vi "Handle Command.vi"(8 "error in (no error)":errorcluster, 9 "Data":variant, 10 "Command":string, 11 "Instrument in":refnum<class "Instrument.lvclass">) -> (0 "error out":errorcluster, 1 "Processed Data":variant, 2 "Command":string, 3 "Instrument out":refnum<class "Instrument.lvclass">)   [LabVIEW 2016, in "Instrument.lvclass"]
uses:
  Instrument.lvclass
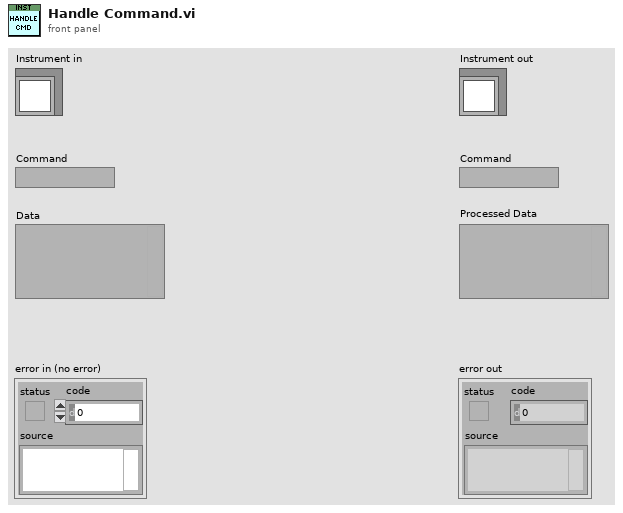
[diagram p1: front panel]
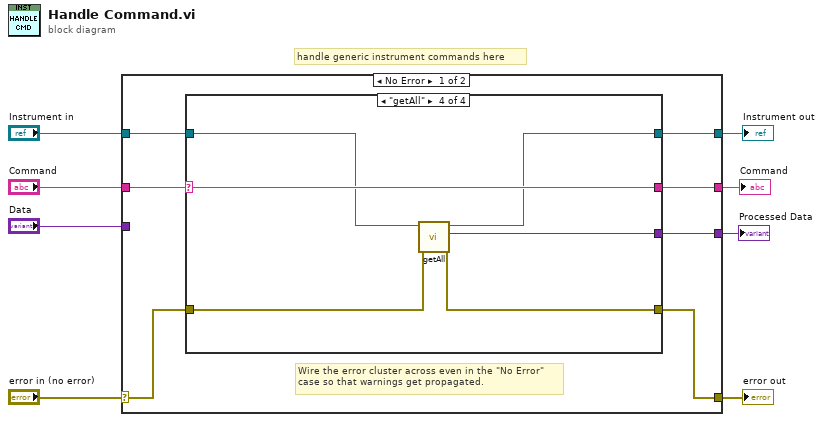
[diagram p0: block diagram]
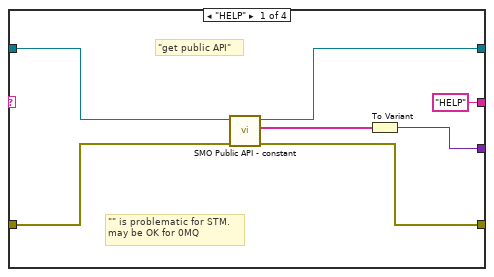
[diagram p2: hidden frame]
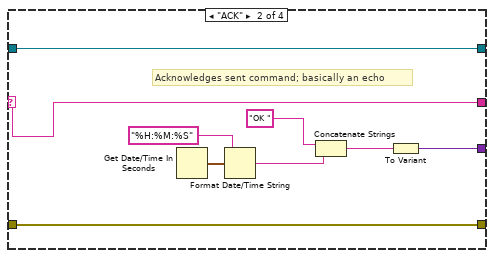
[diagram p3: hidden frame]
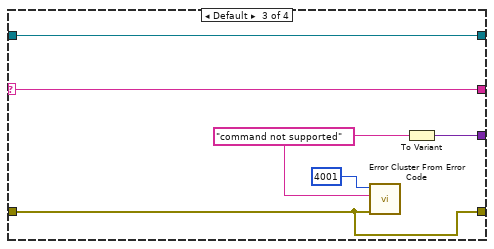
[diagram p4: hidden frame]
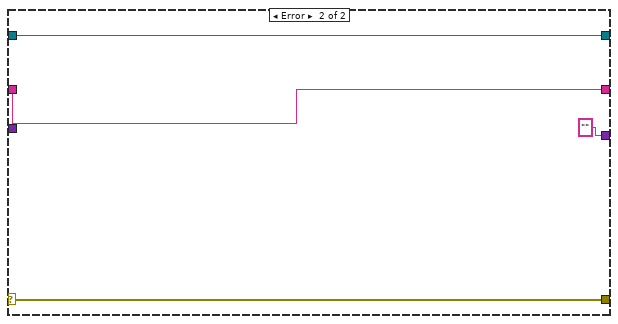
[diagram p5: hidden frame]
diagram:
  # "handle generic instrument commands here"
  n1 = case shown="No Error" "error in (no error)" {
    selector: "error in (no error)" -> [w12 w47]
    tunnel: [w11 w47] -> w7
    tunnel: [w14 w46] -> w5
    tunnel: "Instrument in" -> [w15 w46]
    tunnel: "Command" -> [w9 w44]
    tunnel: [w13 "" ("error message (\"\")")] -> w4
    tunnel: "Data" -> [_ _]
    tunnel: [w10 w44] -> w1
    frame No Error {
      # "Wire the error cluster across even in the \"No Error\"\ncase so that warnings get propagated."
      n2 = case shown="\"getAll\"" w9 {
        selector: w9 -> [_ w23 w33 w43]
        tunnel: w15 -> [w22 w31 w37 w39]
        tunnel: [w20 w31 w37 w38] -> w14
        tunnel: [w18 w24 w34 w42] -> w13
        tunnel: w12 -> [w21 w27 w36 w41]
        tunnel: [w19 w27 w36 w40] -> w11
        tunnel: ["HELP" w23 w33 w43] -> w10
        frame "HELP" {
          # "\"\" is problematic for STM.\nmay be OK for 0MQ"
          # "\"get public API\""
          n3 = call-dynamic "SMO Public API - constant.vi"("error in (no error)"=w21, "Instrument in"=w22) -> ("error out"=w19:errorcluster, "Commands"=w17:string[], "Instrument out"=w20:refnum<class "Instrument.lvclass">)  [unwired: 7 in]
          n4 = To Variant(anything=w17) -> (Variant=w18:variant)
        }
        frame "ACK" {
          # "Acknowledges sent command; basically an echo"
          n5 = Get Date/Time In Seconds() -> (seconds since 1Jan1904=w28:timestamp)
          n6 = Format Date/Time String(time format string (%c)="%H:%M:%S", seconds (now)=w28) -> (date/time string=w29:string)  [unwired: 1 in]
          n7 = Concatenate Strings("OK " ("data"), w29) -> (w26:string)
          n8 = To Variant(anything=w26) -> (Variant=w24:variant)
        }
        frame Default {
          w35 = "command not supported" ("error message (\"\")")
          n9 = call <vilib>:"Error Cluster From Error Code.vi"("error in (no error)"=w36, "error message (\"\")"=w35, "error code (0)"=4001) -> ()  [unwired: 6 in, 1 out]
          n10 = To Variant(anything=w35) -> (Variant=w34:variant)
        }
        frame "getAll" {
          n11 = call-dynamic "getAll.vi"("error in (no error)"=w41, "Instrument in"=w39) -> ("error out"=w40:errorcluster, "getAll"=w42:variant, "Instrument out"=w38:refnum<class "Instrument.lvclass">)  [unwired: 7 in]
        }
      }
    }
    frame Error {
    }
  }
  "error out" <- w7
  "Instrument out" <- w5
  "Processed Data" <- w4
  "Command" <- w1
